vi "LightUpGameboard Test.vi"() -> ()   [LabVIEW 2020]
uses:
  controls/keyboard 3x3.ctl
panel:
  in  "Indices":i8[](array[numeric])
  in  "Gameboard":T1
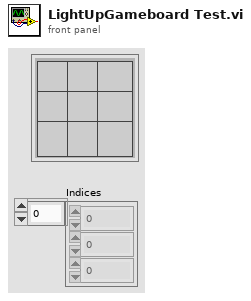
[diagram p1: front panel]
types:
  T1 = typedef "keyboard 3x3.ctl" = cluster{"Button 1":bool, "Button 2":bool, "Button 3":bool, "Button 4":bool, "Button 5":bool, "Button 6":bool, "Button 7":bool, "Button 8":bool, "Button 9":bool}
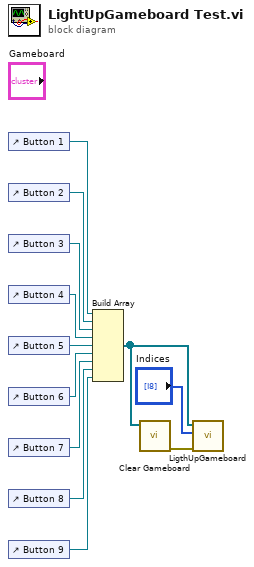
[diagram p0: block diagram]
diagram:
  n1 = control-ref of="Button 1"() -> (w12:refnum<vi>)
  n2 = control-ref of="Button 2"() -> (w11:refnum<vi>)
  n3 = control-ref of="Button 3"() -> (w10:refnum<vi>)
  n4 = control-ref of="Button 4"() -> (w9:refnum<vi>)
  n5 = control-ref of="Button 5"() -> (w8:refnum<vi>)
  n6 = control-ref of="Button 6"() -> (w7:refnum<vi>)
  n7 = control-ref of="Button 7"() -> (w6:refnum<vi>)
  n8 = control-ref of="Button 8"() -> (w5:refnum<vi>)
  n9 = control-ref of="Button 9"() -> (w4:refnum<vi>)
  n10 = Build Array(w12, w11, w10, w9, w8, w7, w6, w5, w4) -> (w2:refnum<vi>[])
  n11 = call "Clear Gameboard.vi"("Buton Refs IN"=w2) -> ("error out"=w1:errorcluster)  [unwired: 9 in, 1 out]
  n12 = call "LigthUpGameboard.vi"("error in (no error)"=w1, "Indices"="Indices", "Button Refs"=w2) -> ()  [unwired: 8 in, 1 out]
